vi "Append Watermark Image.vi"(0 "PDF Report IN":T22(xcontrol), 2 "Watermark Image":T1={"Image path"=path "", "Opacity (%)"=10.0, "Postion"={"Position"=enum."Center (text section)", "X"=0.0, "Y"=0.0}, "Automatic"=FALSE, "Scale(%)"=100.0, "Rotate(°)"=0.0}, 11 "error in (no error)":errorcluster) -> (4 "PDF Report OUT":T22(xcontrol), 15 "error out":errorcluster)   [LabVIEW 2012]
doc: "Appends a <B>watermark</B> (text or image) on each page of the PDF report. \n\n<B>FRANÇAIS</B>\nAjoute un <B>filigrane</B> (texte or image) sur chaque page du rapport PDF. \n\nVersion 1.0\nDeveloped by Jean-Marc Simard\nCopyright © 2010, Exaprom Inc.\nAll rights reserved.\nLicense: BSD\n\nWith iTextSharp Library\n(http://itextsharp.sourceforge.net)"
uses:
  Controls/Font color.ctl
  Controls/Font size.ctl
  Controls/Font cluster.ctl
  C:/Users/MaxCorp/Documents/GitHub/TopView/DLL/itextsharp.dll
  GitHub/TopView/DLL/itextsharp.dll
  Controls/Header footer horiz alignment.ctl
  Controls/PDF Report Xcontrol/PDF Report.xctl
  Controls/Watermark Position.ctl
  Controls/Watermark Image Cluster.ctl
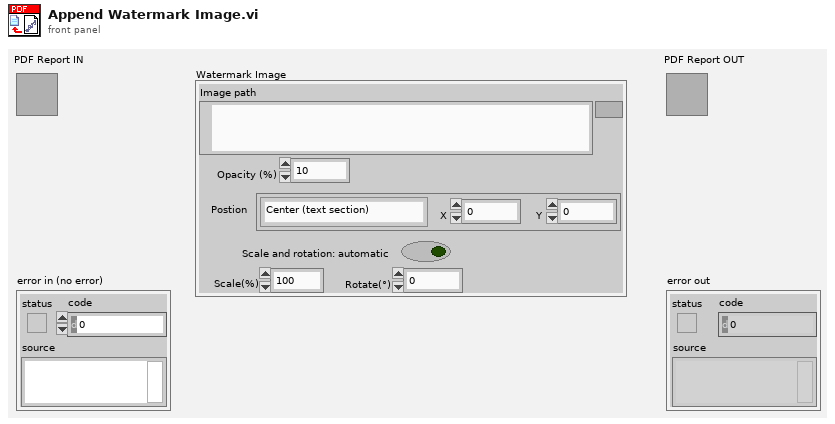
[diagram p1: front panel]
types:
  T1 = typedef "Watermark Image Cluster.ctl" = cluster{"Image path":path, "Opacity (%)":sgl, "Postion":cluster{"Position":T2, "X":sgl, "Y":sgl}, "Automatic":bool, "Scale(%)":sgl, "Rotate(°)":sgl}
  T2 = typedef "Watermark Position.ctl" = enum16{"Absolute", "Center (page)", "Center (text section)"}
  T3 = typedef "Font cluster.ctl" = cluster{"Name":string, "Size":T4, "Color":T5, "Style":cluster{"Bold":bool, "Italic":bool, "Underline":bool, "Strikeout":bool}}
  T4 = typedef "Font size.ctl" = sgl
  T5 = typedef "Font color.ctl" = u32
  T6 = typedef "Unit.ctl" = enum16{"inch", "mm"}
  T7 = typedef "Paragraphe cluster.ctl" = cluster{" Aligment":T8, "Line spacing":T9}
  T8 = typedef "Texte alignement.ctl" = enum16{"Select", "CENTER", "JUSTIFY", "LEFT", "RIGHT"}
  T9 = typedef "Line spacing.ctl" = enum16{"Select", "1.0", "1.5", "2.0"}
  T10 = typedef "Page dimensions.ctl" = cluster{"Start at page":i32, "Orientation":T11, "widht":sgl, "height":sgl, "Margin left":sgl, "Margin right":sgl, "Margin top":sgl, "Margin bottom":sgl}
  T11 = typedef "Page Orientation.ctl" = enum16{"Portrait", "Landscape"}
  T12 = typedef "Image or Table Caption.ctl" = cluster{"Caption":string, "Separator":string, "Position":enum16{"Above", "Below"}}
  T13 = typedef "Header Footer [ ].ctl" = T14[]
  T14 = typedef "Header Footer cluster.ctl" = cluster{"Start page":i32, "Type":T15, "Alignment":T16, "Vertical Alignement":T17, "Image (%)":sgl, "Page #":T18, "Text":string, "Path":string, "Font":T3, "Font refnum":refnum<k24>, "Line":cluster{"Line":T19, "Thickness (points)":sgl, "Colour":T5}}
  T15 = typedef "Header Footer Type.ctl" = enum16{"Select", "Text", "Text + hyperlink", "Page number", "Image", "Image + hyperlink"}
  T16 = typedef "Header footer horiz alignment.ctl" = enum16{"Left", "Center", "Right"}
  T17 = typedef "Cell Vertical alignment.ctl" = enum16{"TOP", "MIDDLE", "BOTTOM"}
  T18 = typedef "Page number.ctl" = cluster{"Text 1":string, "Text 2":string, "Text 3":string}
  T19 = typedef "Header Footer Line.ctl" = enum16{"No line", "Horizontal line"}
  T20 = typedef "Watermark cluster2.ctl" = cluster{"Show? (F)":bool, "Type":enum16{"Image", "Text"}, "Opacity (%)":sgl, "Rotate(°)":sgl, "Position":cluster{"Position":T2, "X":sgl, "Y":sgl}, "Image path":path, "Scaled(%)":sgl, "Image refnum":refnum<k24>, "Text":string, "Font":cluster{"Name":string, "Size":T4, "Color":T5}, "Font refnum":refnum<k24>, "Alignment":T16, "Automatic":bool}
  T21 = typedef "System Fonts.ctl" = cluster{"Font name [ ]":string[], "Font and file names [ ]":cluster{"Font name":string, "File name":string}[]}
  T22 = cluster{"Document":refnum<k24>, "Writer":refnum<k24>, "Default Font":refnum<k24>, "Default Font cluster":T3, "Path":path, "Unit (default = mm)":T6, "Paragraphe cluster":T7, "Pages dimensions [ ]":T10[], "Captions":cluster{"Image":T12, "Image counter":u16, "Table":T12, "Table counter":u16, "Font":T3}, "Header":T13, "Footer":T13, "Watermark ":T20, "Actual VI name":string, "System Fonts":T21}
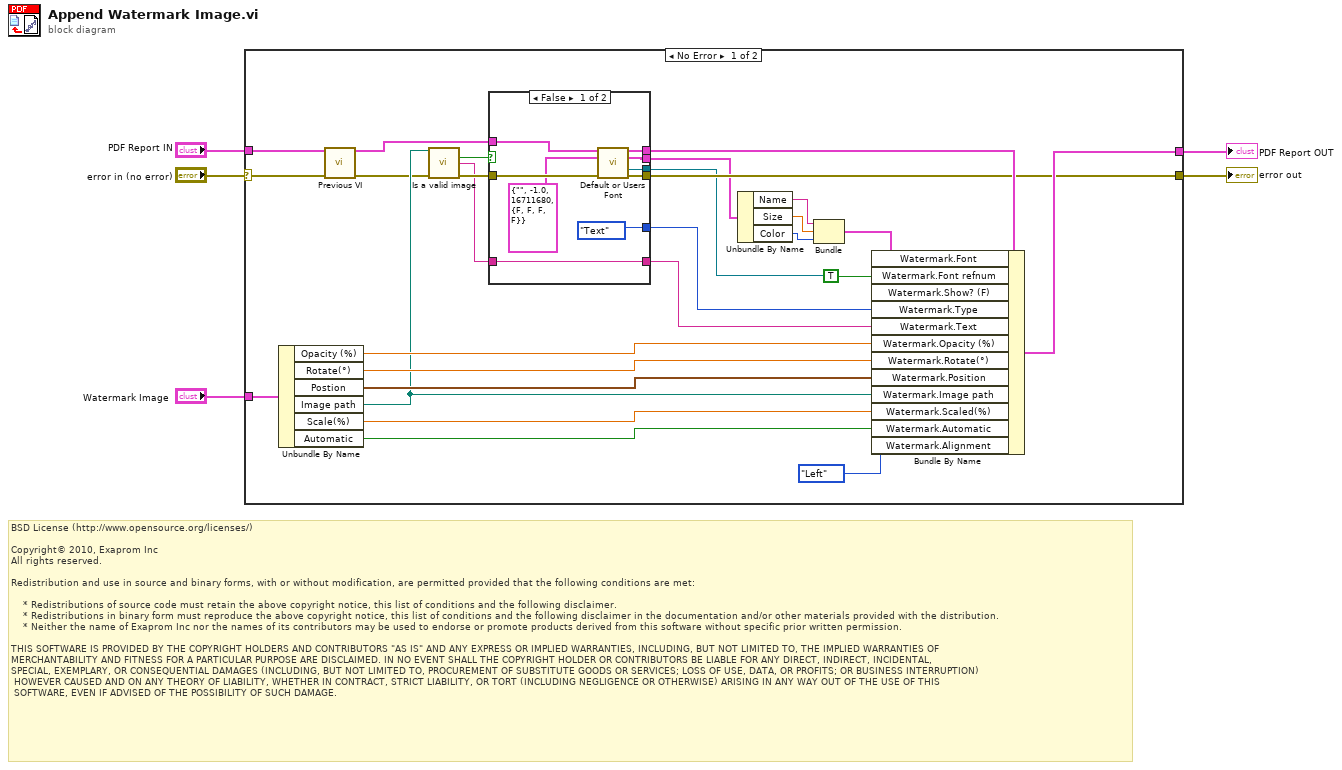
[diagram p0: block diagram]
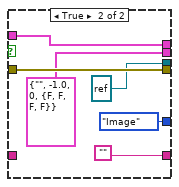
[diagram p2: hidden frame]
diagram:
  # "BSD License (http://www.opensource.org/licenses/)\n\nCopyright© 2010, Exaprom Inc\nAll rights reserved.\n\nRedistribution and use in source and binary forms, with or without modification, are permitted provided that the following conditions are met:\n\n    * Redistributions of source code must retain the above copyright notice, this list of conditions and the following disclaimer.\n    * Redistributions in binary form must reproduce the above copyright notice, this list of conditions and the following disclaimer in the documentation and/or other materials provided with the distribution.\n    * Neither the name of Exaprom Inc nor the names of its contributors may be used to endorse or promote products derived from this software without specific prior written permission.\n\nTHIS SOFTWARE IS PROVIDED BY THE COPYRIGHT HOLDERS AND CONTRIBUTORS \"AS IS\" AND ANY EXPRESS OR IMPLIED WARRANTIES, INCLUDING, BUT NOT LIMITED TO, THE IMPLIED WARRANTIES OF \nMERCHANTABILITY AND FITNESS FOR A PARTICULAR PURPOSE ARE DISCLAIMED. IN NO EVENT SHALL THE COPYRIGHT HOLDER OR CONTRIBUTORS BE LIABLE FOR ANY DIRECT, INDIRECT, INCIDENTAL,\nSPECIAL, EXEMPLARY, OR CONSEQUENTIAL DAMAGES (INCLUDING, BUT NOT LIMITED TO, PROCUREMENT OF SUBSTITUTE GOODS OR SERVICES; LOSS OF USE, DATA, OR PROFITS; OR BUSINESS INTERRUPTION)\n HOWEVER CAUSED AND ON ANY THEORY OF LIABILITY, WHETHER IN CONTRACT, STRICT LIABILITY, OR TORT (INCLUDING NEGLIGENCE OR OTHERWISE) ARISING IN ANY WAY OUT OF THE USE OF THIS\n SOFTWARE, EVEN IF ADVISED OF THE POSSIBILITY OF SUCH DAMAGE."
  n1 = case shown="No Error" "error in (no error)" {
    selector: "error in (no error)" -> [w30 w49]
    tunnel: "PDF Report IN" -> [w31 w48]
    tunnel: "Watermark Image" -> [w29 _]
    tunnel: [w32 w48] -> w3
    tunnel: [w14 w49] -> w2
    frame No Error {
      n2 = Unbundle By Name(w29) -> ("Opacity (%)"=w28:sgl, "Rotate(°)"=w27:sgl, "Postion"=w26:cluster{"Position":T2, "X":sgl, "Y":sgl}, "Image path"=w18:path, "Scale(%)"=w25:sgl, "Automatic"=w23:bool)
      n3 = call "Previous VI.vi"("PDF Report IN"=w31, "error in (no error)"=w30) -> ("PDF Report OUT"=w17:T22, "error out"=w15:errorcluster)  [unwired: 12 out]
      n4 = call "Is a valid image.vi"("Image path"=w18, "error in (no error)"=w15) -> ("Valid Image?"=w19:bool, "Message"=w20:string, "error out"=w21:errorcluster)  [unwired: 11 out]
      n5 = case shown="False" w19 {
        tunnel: [enum16{"Image", "Text"}."Text" ("Watermark .Type") enum16{"Image", "Text"}."Image" ("Watermark .Type")] -> w8
        tunnel: [w41 ""] -> w7
        tunnel: w20 -> [w41 _]
        tunnel: [w39 w47] -> w16
        tunnel: w17 -> [w40 w47]
        tunnel: w21 -> [w38 w46]
        tunnel: [w37 T3 {"Name"="", "Size"=-1.0, "Color"=0, "Style"={"Bold"=FALSE, "Italic"=FALSE, "Underline"=FALSE, "Strikeout"=FALSE}} ("Font OUT")] -> w13
        tunnel: [w36 refnum<k24> refnum ("Font Ref")] -> w9
        tunnel: [w35 w46] -> w14
        frame False {
          n6 = call "Default or Users Font.vi"("PDF Report"=w40, "Font"=T3 {"Name"="", "Size"=-1.0, "Color"=16711680, "Style"={"Bold"=FALSE, "Italic"=FALSE, "Underline"=FALSE, "Strikeout"=FALSE}} ("Font OUT"), "error in (no error)"=w38) -> ("PDF Report duplicate"=w39:T22, "Font OUT"=w37:T3, "Font Ref"=w36:refnum<k24>, "error out"=w35:errorcluster)  [unwired: 9 out]
        }
        frame True {
        }
      }
      n7 = Unbundle By Name(w13) -> ("Name"=w12:string, "Size"=w11:T4, "Color"=w10:T5)
      n8 = Bundle("Name"=w12, "Size"=w11, "Color"=w10) -> (w22:cluster{"Name":string, "Size":T4, "Color":T5})  [unwired: 1 out]
      n9 = Bundle By Name(cluster=w16, "Watermark.Font"=w22, "Watermark.Font refnum"=w9, "Watermark.Show? (F)"=TRUE ("Watermark .Show? (F)"), "Watermark.Type"=w8, "Watermark.Text"=w7, "Watermark.Opacity (%)"=w28, "Watermark.Rotate(°)"=w27, "Watermark.Position"=w26, "Watermark.Image path"=w18, "Watermark.Scaled(%)"=w25, "Watermark.Automatic"=w23, "Watermark.Alignment"=Header_footer_horiz_alignment."Left" ("Watermark .Alignment")) -> (w32:T22)
    }
    frame Error {
    }
  }
  "PDF Report OUT" <- w3
  "error out" <- w2
